vi "Describe String Failure.vi"(1 "Expected":string, 2 "Got":string) -> (0 "Failure Description":string)   [LabVIEW 2013]
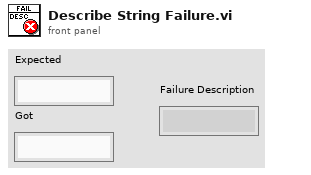
[diagram p1: front panel]
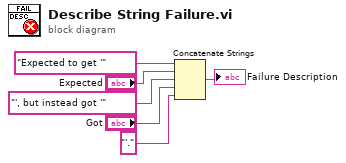
[diagram p0: block diagram]
diagram:
  n1 = Concatenate Strings("Expected to get '", "Expected", "', but instead got '", "Got", "'.") -> (→"Failure Description":string)
